vi "Generate waveform.vi"(8 "error in (no error)":errorcluster, 11 "Galvo in":refnum<class "InVivo_ImagingModeSPIM.lvclass">) -> (0 "error out":errorcluster, 2 "Array":variant[](array[variant]), 3 "Galvo out":refnum<class "InVivo_ImagingModeSPIM.lvclass">)   [LabVIEW 2012, in "InVivo_ImagingModeSPIM.lvclass"]
uses:
  InVivo_ImagingModeSPIM.lvclass
  InVivo_ImagingModeSPIM.lvclass/InVivo_ImagingModeSPIM.ctl
  <vilib>/measure/NI_MABase.lvlib
panel:
  out "Waveformvalues":variant
  out "Mixed Signal Graph 2":waveform(dbl)(graph)
  out "Mixed Signal Graph":waveform(dbl)[](graph)
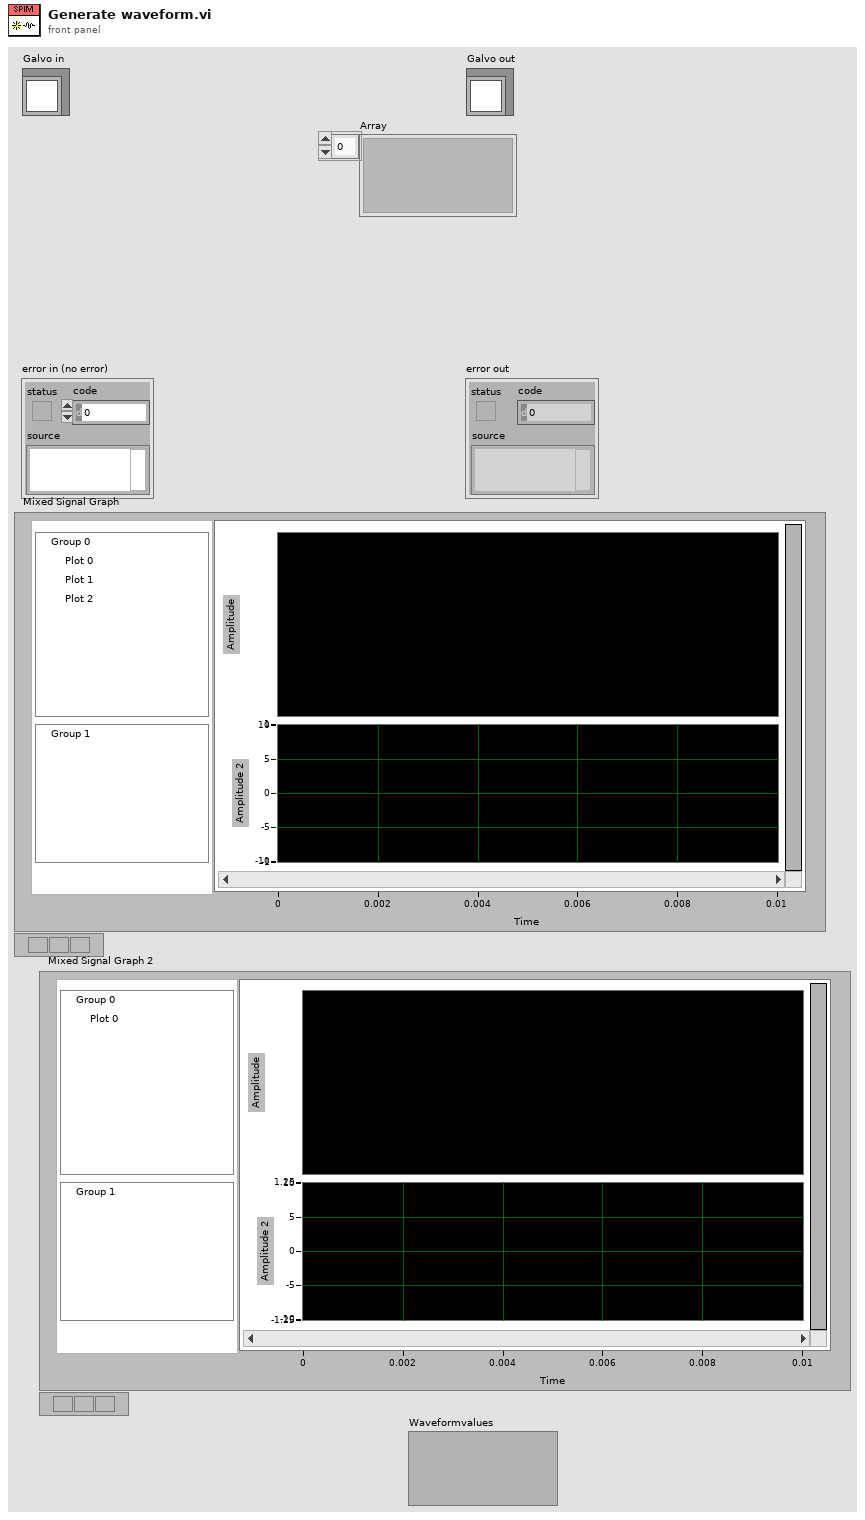
[diagram p1: front panel]
types:
  T1 = typedef "InVivo_ImagingModeSPIM.lvclass/waveform_enum.ctl" = enum16{"triangular", "sawtooth", "sinusodial"}
  T2 = typedef "InVivo_ImagingModeSPIM.lvclass/Control 4.ctl" = enum16{"Triangular", "Sawtooth", "Sinusoidal"}
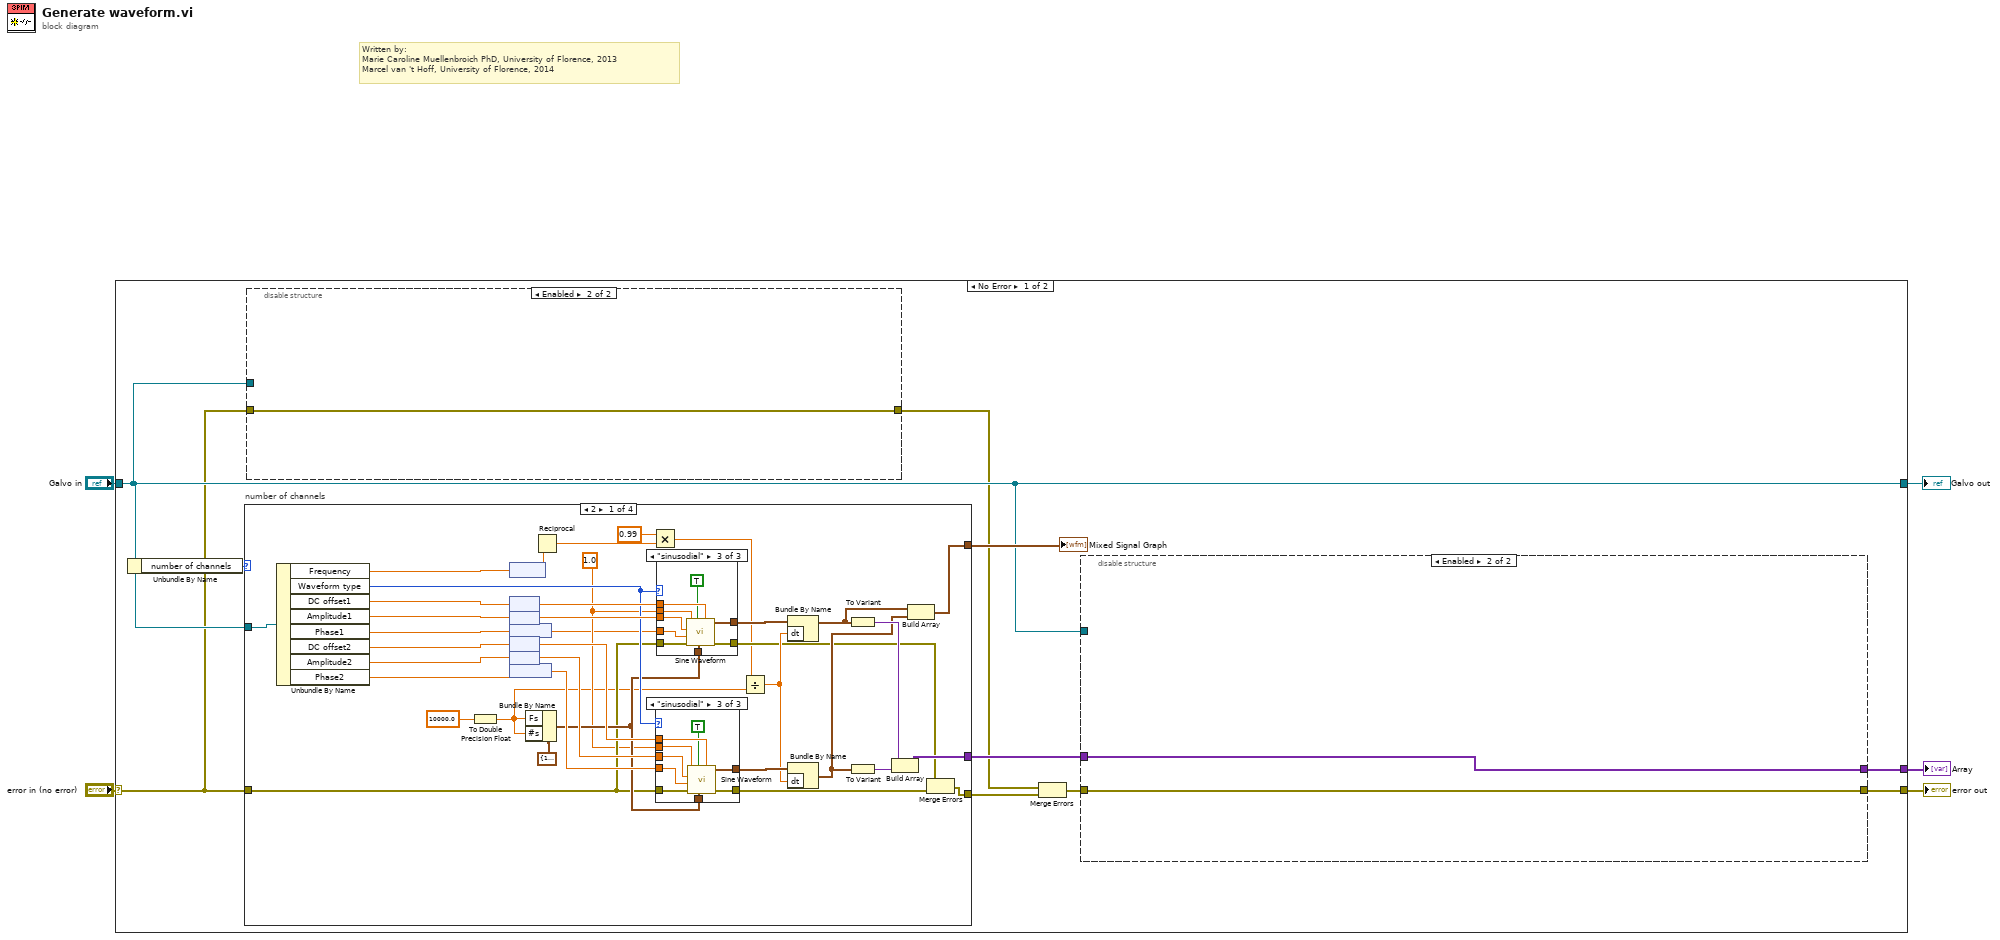
[diagram p0: block diagram]
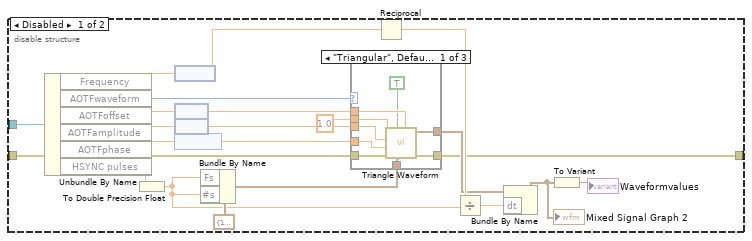
[diagram p2: hidden frame]
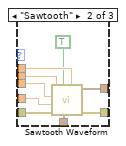
[diagram p3: hidden frame]
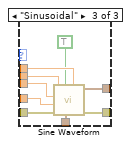
[diagram p4: hidden frame]
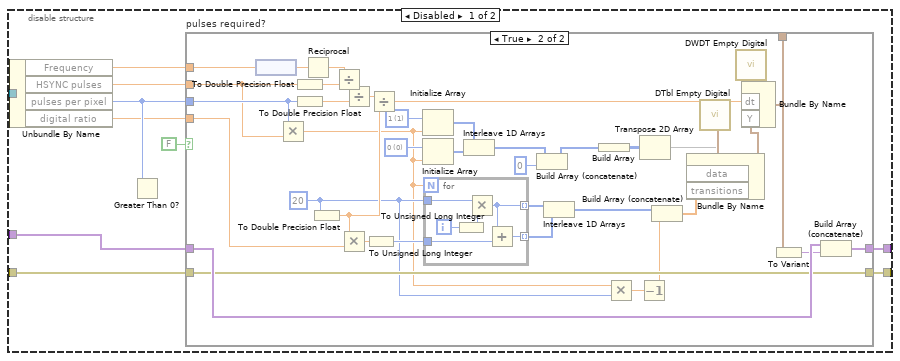
[diagram p5: hidden frame]
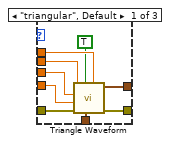
[diagram p7: hidden frame]
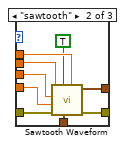
[diagram p8: hidden frame]
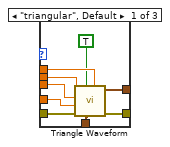
[diagram p9: hidden frame]
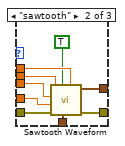
[diagram p10: hidden frame]
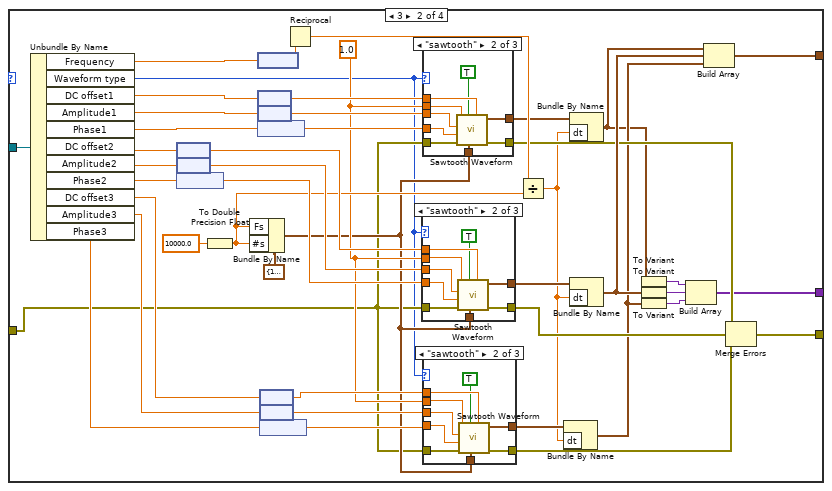
[diagram p11: hidden frame]
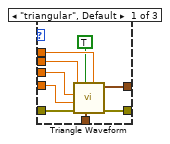
[diagram p12: hidden frame]
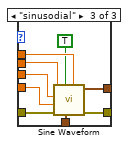
[diagram p13: hidden frame]
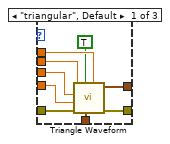
[diagram p14: hidden frame]
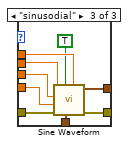
[diagram p15: hidden frame]
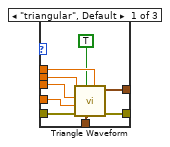
[diagram p16: hidden frame]
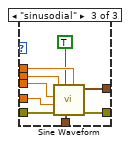
[diagram p17: hidden frame]
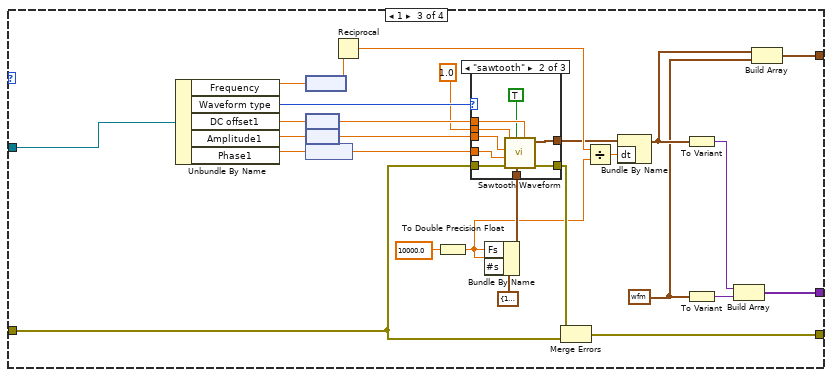
[diagram p18: hidden frame]
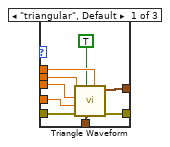
[diagram p19: hidden frame]
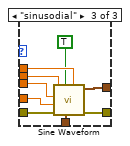
[diagram p20: hidden frame]
diagram:
  # "Written by:\nMarie Caroline Muellenbroich PhD, University of Florence, 2013 \nMarcel van 't Hoff, University of Florence, 2014"
  n1 = case shown="No Error" "error in (no error)" {
    selector: "error in (no error)" -> [w9 w398]
    tunnel: [w13 w398] -> w5
    tunnel: [w10 w397] -> w4
    tunnel: "Galvo in" -> [w10 w397]
    tunnel: [w15 _] -> w3
    frame No Error {
      n2 = Unbundle By Name(w10) -> ("number of channels"=w12:u8)
      n3 = case "number of channels" shown="2" w12 {
        tunnel: [w146 w223 w360 w396] -> w8
        tunnel: w9 -> [w147 w219 w346 w396]
        tunnel: [w145 w221 w359 _] -> w14
        tunnel: [w132 w222 w349 _] -> w11
        tunnel: w10 -> [w129 w220 w344 _]
        frame 2 {
          w141 = 1.0
          n4 = Unbundle By Name(w129) -> ("Frequency"=w138:dbl[unit], "Waveform type"=w155:T1, "DC offset1"=w156:dbl[unit], "Amplitude1"=w157:dbl[unit], "Phase1"=w158:dbl[unit], "DC offset2"=w153:dbl[unit], "Amplitude2"=w152:dbl[unit], "Phase2"=w151:dbl[unit])
          n5 = To Double Precision Float(number=10000.0) -> (double precision float=w136:dbl)
          n6 = node(w138) -> (w140:dbl)
          n7 = node(w156) -> (w160:dbl)
          n8 = node(w157) -> (w161:dbl)
          n9 = node(w158) -> (w137:dbl)
          n10 = node(w153) -> (w154:dbl)
          n11 = node(w152) -> (w149:dbl)
          n12 = node(w151) -> (w150:dbl)
          n13 = Bundle By Name(cluster=cluster{"Fs":dbl, "#s":dbl} {"Fs"=1000.0, "#s"=1000.0} ("sampling info"), "Fs"=w136, "#s"=w136) -> (w148:cluster{"Fs":dbl, "#s":dbl})
          n14 = Reciprocal(x=w140) -> (1/x=w127:dbl)
          n15 = Multiply(x=0.99, y=w127) -> (x*y=w126:dbl)
          n16 = case shown="\"sinusodial\"" w155 {
            tunnel: w154 -> [w168 w179 w188]
            tunnel: w141 -> [w167 w178 w187]
            tunnel: w148 -> [w169 w177 w186]
            tunnel: [w166 w176 w185] -> w139
            tunnel: [w170 w171 w180] -> w142
            tunnel: w149 -> [w163 w174 w183]
            tunnel: w150 -> [w164 w173 w182]
            tunnel: w147 -> [w162 w172 w181]
            frame "triangular", Default {
              n17 = call <vilib>:"Triangle Waveform.vi"("offset"=w168, "sampling info"=w169, "reset signal"=TRUE, "error in (no error)"=w162, "phase"=w164, "amplitude"=w163, "frequency"=w167) -> ("error out"=w170:errorcluster, "signal out"=w166:waveform(dbl))  [unwired: 3 in]
            }
            frame "sawtooth" {
              n18 = call <vilib>:"Sawtooth Waveform.vi"("offset"=w179, "sampling info"=w177, "reset signal"=TRUE, "error in (no error)"=w172, "phase"=w173, "amplitude"=w174, "frequency"=w178) -> ("error out"=w171:errorcluster, "signal out"=w176:waveform(dbl))  [unwired: 3 in]
            }
            frame "sinusodial" {
              n19 = call <vilib>:"Sine Waveform.vi"("offset"=w188, "sampling info"=w186, "reset signal"=TRUE, "error in (no error)"=w181, "phase"=w182, "amplitude"=w183, "frequency"=w187) -> ("error out"=w180:errorcluster, "signal out"=w185:waveform(dbl))  [unwired: 3 in]
            }
          }
          n20 = case shown="\"sinusodial\"" w155 {
            tunnel: w160 -> [w195 w206 w215]
            tunnel: w141 -> [w194 w205 w214]
            tunnel: w161 -> [w193 w204 w213]
            tunnel: w137 -> [w192 w203 w212]
            tunnel: w148 -> [w196 w202 w211]
            tunnel: [w191 w201 w210] -> w133
            tunnel: [w197 w200 w209] -> w130
            tunnel: w147 -> [w189 w198 w207]
            frame "triangular", Default {
              n21 = call <vilib>:"Triangle Waveform.vi"("offset"=w195, "sampling info"=w196, "reset signal"=TRUE, "error in (no error)"=w189, "phase"=w192, "amplitude"=w193, "frequency"=w194) -> ("error out"=w197:errorcluster, "signal out"=w191:waveform(dbl))  [unwired: 3 in]
            }
            frame "sawtooth" {
              n22 = call <vilib>:"Sawtooth Waveform.vi"("offset"=w206, "sampling info"=w202, "reset signal"=TRUE, "error in (no error)"=w198, "phase"=w203, "amplitude"=w204, "frequency"=w205) -> ("error out"=w200:errorcluster, "signal out"=w201:waveform(dbl))  [unwired: 3 in]
            }
            frame "sinusodial" {
              n23 = call <vilib>:"Sine Waveform.vi"("offset"=w215, "sampling info"=w211, "reset signal"=TRUE, "error in (no error)"=w207, "phase"=w212, "amplitude"=w213, "frequency"=w214) -> ("error out"=w209:errorcluster, "signal out"=w210:waveform(dbl))  [unwired: 3 in]
            }
          }
          n24 = Divide(x=w126, y=w136) -> (x/y=w135:dbl)
          n25 = Bundle By Name(cluster=w133, "dt"=w135) -> (w131:waveform(dbl))
          n26 = Bundle By Name(cluster=w139, "dt"=w135) -> (w134:waveform(dbl))
          n27 = To Variant(anything=w131) -> (Variant=w143:variant)
          n28 = To Variant(anything=w134) -> (Variant=w144:variant)
          n29 = Build Array(w143, w144) -> (w145:variant[])
          n30 = Build Array(w131, w134) -> (w132:waveform(dbl)[])
          n31 = Merge Errors(w130, w142) -> (w146:errorcluster)
        }
        frame 3 {
          w230 = 1.0
          n32 = Unbundle By Name(w220) -> ("Frequency"=w243:dbl[unit], "Waveform type"=w218:T1, "DC offset1"=w255:dbl[unit], "Amplitude1"=w256:dbl[unit], "Phase1"=w257:dbl[unit], "DC offset2"=w253:dbl[unit], "Amplitude2"=w252:dbl[unit], "Phase2"=w251:dbl[unit], "DC offset3"=w236:dbl[unit], "Amplitude3"=w235:dbl[unit], "Phase3"=w234:dbl[unit])
          n33 = node(w253) -> (w254:dbl)
          n34 = node(w252) -> (w249:dbl)
          n35 = node(w251) -> (w250:dbl)
          n36 = To Double Precision Float(number=10000.0) -> (double precision float=w241:dbl)
          n37 = Bundle By Name(cluster=cluster{"Fs":dbl, "#s":dbl} {"Fs"=1000.0, "#s"=1000.0} ("sampling info"), "Fs"=w241, "#s"=w241) -> (w229:cluster{"Fs":dbl, "#s":dbl})
          n38 = node(w243) -> (w245:dbl)
          n39 = node(w255) -> (w259:dbl)
          n40 = node(w256) -> (w260:dbl)
          n41 = node(w257) -> (w242:dbl)
          n42 = node(w236) -> (w233:dbl)
          n43 = node(w235) -> (w232:dbl)
          n44 = node(w234) -> (w231:dbl)
          n45 = Reciprocal(x=w245) -> (1/x=w240:dbl)
          n46 = case shown="\"sawtooth\"" w218 {
            tunnel: w254 -> [w294 w305 w314]
            tunnel: w230 -> [w293 w304 w313]
            tunnel: w229 -> [w295 w303 w312]
            tunnel: [w292 w302 w311] -> w244
            tunnel: [w296 w297 w306] -> w246
            tunnel: w249 -> [w289 w300 w309]
            tunnel: w250 -> [w290 w299 w308]
            tunnel: w219 -> [w288 w298 w307]
            frame "triangular", Default {
              n47 = call <vilib>:"Triangle Waveform.vi"("offset"=w294, "sampling info"=w295, "reset signal"=TRUE, "error in (no error)"=w288, "phase"=w290, "amplitude"=w289, "frequency"=w293) -> ("error out"=w296:errorcluster, "signal out"=w292:waveform(dbl))  [unwired: 3 in]
            }
            frame "sawtooth" {
              n48 = call <vilib>:"Sawtooth Waveform.vi"("offset"=w305, "sampling info"=w303, "reset signal"=TRUE, "error in (no error)"=w298, "phase"=w299, "amplitude"=w300, "frequency"=w304) -> ("error out"=w297:errorcluster, "signal out"=w302:waveform(dbl))  [unwired: 3 in]
            }
            frame "sinusodial" {
              n49 = call <vilib>:"Sine Waveform.vi"("offset"=w314, "sampling info"=w312, "reset signal"=TRUE, "error in (no error)"=w307, "phase"=w308, "amplitude"=w309, "frequency"=w313) -> ("error out"=w306:errorcluster, "signal out"=w311:waveform(dbl))  [unwired: 3 in]
            }
          }
          n50 = case shown="\"sawtooth\"" w218 {
            tunnel: w259 -> [w321 w332 w341]
            tunnel: w230 -> [w320 w331 w340]
            tunnel: w260 -> [w319 w330 w339]
            tunnel: w242 -> [w318 w329 w338]
            tunnel: w229 -> [w322 w328 w337]
            tunnel: [w317 w327 w336] -> w238
            tunnel: [w323 w326 w335] -> w237
            tunnel: w219 -> [w315 w324 w333]
            frame "triangular", Default {
              n51 = call <vilib>:"Triangle Waveform.vi"("offset"=w321, "sampling info"=w322, "reset signal"=TRUE, "error in (no error)"=w315, "phase"=w318, "amplitude"=w319, "frequency"=w320) -> ("error out"=w323:errorcluster, "signal out"=w317:waveform(dbl))  [unwired: 3 in]
            }
            frame "sawtooth" {
              n52 = call <vilib>:"Sawtooth Waveform.vi"("offset"=w332, "sampling info"=w328, "reset signal"=TRUE, "error in (no error)"=w324, "phase"=w329, "amplitude"=w330, "frequency"=w331) -> ("error out"=w326:errorcluster, "signal out"=w327:waveform(dbl))  [unwired: 3 in]
            }
            frame "sinusodial" {
              n53 = call <vilib>:"Sine Waveform.vi"("offset"=w341, "sampling info"=w337, "reset signal"=TRUE, "error in (no error)"=w333, "phase"=w338, "amplitude"=w339, "frequency"=w340) -> ("error out"=w335:errorcluster, "signal out"=w336:waveform(dbl))  [unwired: 3 in]
            }
          }
          n54 = case shown="\"sawtooth\"" w218 {
            tunnel: w233 -> [w267 w278 w287]
            tunnel: w230 -> [w266 w277 w286]
            tunnel: w229 -> [w268 w276 w285]
            tunnel: [w265 w275 w284] -> w228
            tunnel: [w269 w270 w279] -> w227
            tunnel: w232 -> [w262 w273 w282]
            tunnel: w231 -> [w263 w272 w281]
            tunnel: w219 -> [w261 w271 w280]
            frame "triangular", Default {
              n55 = call <vilib>:"Triangle Waveform.vi"("offset"=w267, "sampling info"=w268, "reset signal"=TRUE, "error in (no error)"=w261, "phase"=w263, "amplitude"=w262, "frequency"=w266) -> ("error out"=w269:errorcluster, "signal out"=w265:waveform(dbl))  [unwired: 3 in]
            }
            frame "sawtooth" {
              n56 = call <vilib>:"Sawtooth Waveform.vi"("offset"=w278, "sampling info"=w276, "reset signal"=TRUE, "error in (no error)"=w271, "phase"=w272, "amplitude"=w273, "frequency"=w277) -> ("error out"=w270:errorcluster, "signal out"=w275:waveform(dbl))  [unwired: 3 in]
            }
            frame "sinusodial" {
              n57 = call <vilib>:"Sine Waveform.vi"("offset"=w287, "sampling info"=w285, "reset signal"=TRUE, "error in (no error)"=w280, "phase"=w281, "amplitude"=w282, "frequency"=w286) -> ("error out"=w279:errorcluster, "signal out"=w284:waveform(dbl))  [unwired: 3 in]
            }
          }
          n58 = Divide(x=w240, y=w241) -> (x/y=w226:dbl)
          n59 = Bundle By Name(cluster=w228, "dt"=w226) -> (w224:waveform(dbl))
          n60 = Bundle By Name(cluster=w238, "dt"=w226) -> (w216:waveform(dbl))
          n61 = Bundle By Name(cluster=w244, "dt"=w226) -> (w239:waveform(dbl))
          n62 = To Variant(anything=w216) -> (Variant=w247:variant)
          n63 = To Variant(anything=w239) -> (Variant=w248:variant)
          n64 = To Variant(anything=w224) -> (Variant=w225:variant)
          n65 = Build Array(w247, w248, w225) -> (w221:variant[])
          n66 = Build Array(w216, w239, w224) -> (w222:waveform(dbl)[])
          n67 = Merge Errors(w237, w246, w227) -> (w223:errorcluster)
        }
        frame 1 {
          w345 = waveform(dbl) {"t0"=timestamp(0 s since 1904-01-01), "dt"=1.0, "Y"=[]} ("signal out")
          n68 = Unbundle By Name(w344) -> ("Frequency"=w354:dbl[unit], "Waveform type"=w362:T1, "DC offset1"=w363:dbl[unit], "Amplitude1"=w364:dbl[unit], "Phase1"=w365:dbl[unit])
          n69 = node(w354) -> (w355:dbl)
          n70 = node(w363) -> (w367:dbl)
          n71 = node(w364) -> (w368:dbl)
          n72 = node(w365) -> (w353:dbl)
          n73 = Reciprocal(x=w355) -> (1/x=w352:dbl)
          n74 = To Double Precision Float(number=10000.0) -> (double precision float=w342:dbl)
          n75 = Bundle By Name(cluster=cluster{"Fs":dbl, "#s":dbl} {"Fs"=10000.0, "#s"=10000.0} ("sampling info"), "Fs"=w342, "#s"=w342) -> (w361:cluster{"Fs":dbl, "#s":dbl})
          n76 = case shown="\"sawtooth\"" w362 {
            tunnel: w367 -> [w375 w386 w395]
            tunnel: 1.0 -> [w374 w385 w394]
            tunnel: w368 -> [w373 w384 w393]
            tunnel: w353 -> [w372 w383 w392]
            tunnel: w361 -> [w376 w382 w391]
            tunnel: [w371 w381 w390] -> w350
            tunnel: [w377 w380 w389] -> w347
            tunnel: w346 -> [w369 w378 w387]
            frame "triangular", Default {
              n77 = call <vilib>:"Triangle Waveform.vi"("offset"=w375, "sampling info"=w376, "reset signal"=TRUE, "error in (no error)"=w369, "phase"=w372, "amplitude"=w373, "frequency"=w374) -> ("error out"=w377:errorcluster, "signal out"=w371:waveform(dbl))  [unwired: 3 in]
            }
            frame "sawtooth" {
              n78 = call <vilib>:"Sawtooth Waveform.vi"("offset"=w386, "sampling info"=w382, "reset signal"=TRUE, "error in (no error)"=w378, "phase"=w383, "amplitude"=w384, "frequency"=w385) -> ("error out"=w380:errorcluster, "signal out"=w381:waveform(dbl))  [unwired: 3 in]
            }
            frame "sinusodial" {
              n79 = call <vilib>:"Sine Waveform.vi"("offset"=w395, "sampling info"=w391, "reset signal"=TRUE, "error in (no error)"=w387, "phase"=w392, "amplitude"=w393, "frequency"=w394) -> ("error out"=w389:errorcluster, "signal out"=w390:waveform(dbl))  [unwired: 3 in]
            }
          }
          n80 = Merge Errors(w347, w346) -> (w360:errorcluster)
          n81 = Divide(x=w352, y=w342) -> (x/y=w351:dbl)
          n82 = Bundle By Name(cluster=w350, "dt"=w351) -> (w348:waveform(dbl))
          n83 = To Variant(anything=w348) -> (Variant=w357:variant)
          n84 = To Variant(anything=w345) -> (Variant=w358:variant)
          n85 = Build Array(w357, w358) -> (w359:variant[])
          n86 = Build Array(w348, w345) -> (w349:waveform(dbl)[])
        }
        frame Default {
        }
      }
      "Mixed Signal Graph" <- w11
      n87 = disable-structure shown="Enabled" {
        disable-tunnel: w10 -> [w37 _]
        disable-tunnel: w9 -> [w36 w65]
        disable-tunnel: [w17 w65] -> w6
        frame Disabled {
          n88 = Unbundle By Name(w37) -> ("Frequency"=w23:dbl[unit], "AOTFwaveform"=w28:T2, "AOTFoffset"=w29:dbl[unit], "AOTFamplitude"=w30:dbl[unit], "AOTFphase"=w31:dbl[unit], "HSYNC pulses"=w27:dbl)
          n89 = To Double Precision Float(number=w27) -> (double precision float=w21:dbl)
          n90 = node(w23) -> (w24:dbl)
          n91 = node(w29) -> (w33:dbl)
          n92 = node(w30) -> (w34:dbl)
          n93 = node(w31) -> (w22:dbl)
          n94 = Bundle By Name(cluster=cluster{"Fs":dbl, "#s":dbl} {"Fs"=1000.0, "#s"=1000.0} ("sampling info"), "Fs"=w21, "#s"=w21) -> (w26:cluster{"Fs":dbl, "#s":dbl})
          n95 = case shown="\"Triangular\", Default" w28 {
            tunnel: w33 -> [w44 w55 w64]
            tunnel: 1.0 -> [w43 w54 w63]
            tunnel: w34 -> [w42 w53 w62]
            tunnel: w22 -> [w41 w52 w61]
            tunnel: w26 -> [w45 w51 w60]
            tunnel: [w40 w50 w59] -> w18
            tunnel: [w46 w49 w58] -> w17
            tunnel: w36 -> [w38 w47 w56]
            frame "Triangular", Default {
              n96 = call <vilib>:"Triangle Waveform.vi"("offset"=w44, "sampling info"=w45, "reset signal"=TRUE, "error in (no error)"=w38, "phase"=w41, "amplitude"=w42, "frequency"=w43) -> ("error out"=w46:errorcluster, "signal out"=w40:waveform(dbl))  [unwired: 3 in]
            }
            frame "Sawtooth" {
              n97 = call <vilib>:"Sawtooth Waveform.vi"("offset"=w55, "sampling info"=w51, "reset signal"=TRUE, "error in (no error)"=w47, "phase"=w52, "amplitude"=w53, "frequency"=w54) -> ("error out"=w49:errorcluster, "signal out"=w50:waveform(dbl))  [unwired: 3 in]
            }
            frame "Sinusoidal" {
              n98 = call <vilib>:"Sine Waveform.vi"("offset"=w64, "sampling info"=w60, "reset signal"=TRUE, "error in (no error)"=w56, "phase"=w61, "amplitude"=w62, "frequency"=w63) -> ("error out"=w58:errorcluster, "signal out"=w59:waveform(dbl))  [unwired: 3 in]
            }
          }
          n99 = Reciprocal(x=w24) -> (1/x=w20:dbl)
          n100 = Divide(x=w20, y=w21) -> (x/y=w19:dbl)
          n101 = Bundle By Name(cluster=w18, "dt"=w19) -> (w16:waveform(dbl))
          "Mixed Signal Graph 2" <- w16
          n102 = To Variant(anything=w16) -> (Variant=→"Waveformvalues":variant)
        }
        frame Enabled {
        }
      }
      n103 = Merge Errors(w6, w8) -> (w7:errorcluster)
      n104 = disable-structure shown="Enabled" {
        disable-tunnel: [w75 w123] -> w15
        disable-tunnel: w14 -> [w74 w123]
        disable-tunnel: [w70 w124] -> w13
        disable-tunnel: w10 -> [w67 _]
        disable-tunnel: w7 -> [w66 w124]
        frame Disabled {
          n105 = Unbundle By Name(w67) -> ("Frequency"=w73:dbl[unit], "HSYNC pulses"=w72:dbl, "pulses per pixel"=w71:i32, "digital ratio"=w69:dbl)
          n106 = Greater Than 0?(x=w71) -> ()  [unwired: 1 out]
          n107 = case "pulses required?" shown="True" FALSE {
            tunnel: w71 -> [_ w81]
            tunnel: [w77 w98] -> w70
            tunnel: w66 -> [w77 w98]
            tunnel: [w76 w111] -> w75
            tunnel: w74 -> [w76 w112]
            tunnel: w73 -> [_ w116]
            tunnel: w72 -> [_ w78]
            tunnel: [_ w108] -> _
            tunnel: w69 -> [_ w94]
            frame False {
            }
            frame True {
              w82 = u32 20 ("ratio step size")
              w100 = u8 0 items=["0", "1", "Z", "L", "H", "X", "T", "V"] ("value 2")
              w99 = u8 1 items=["0", "1", "Z", "L", "H", "X", "T", "V"] ("value 2")
              n108 = node(w116) -> (w115:dbl)
              n109 = Multiply(x=w81, y=w78) -> (x*y=w79:dbl)
              n110 = To Double Precision Float(number=w78) -> (double precision float=w113:dbl)
              n111 = To Double Precision Float(number=w81) -> (double precision float=w109:dbl)
              n112 = Reciprocal(x=w115) -> (1/x=w114:dbl)
              n113 = To Double Precision Float(number=w82) -> (double precision float=w93:dbl)
              n114 = Divide(x=w114, y=w113) -> (x/y=w110:dbl)
              n115 = Multiply(x=w93, y=w94) -> (x*y=w104:dbl)
              n116 = Divide(x=w110, y=w109) -> (x/y=w92:dbl)
              n117 = To Unsigned Long Integer(number=w104) -> (unsigned 32bit integer=w107:u32)
              n118 = Divide(x=w92, y=w93) -> (x/y=w91:dbl)
              n119 = Initialize Array(w99, w79) -> (w102:u8[])
              n120 = Initialize Array(w100, w79) -> (w103:u8[])
              n121 = for {
                N: w79 -> [_]
                tunnel: w107 -> [w120]
                tunnel: w82 -> [w122]
                tunnel: [w119] -> w105 mode=indexing
                tunnel: [w118] -> w106 mode=indexing
                i -> [w121]
                n122 = To Unsigned Long Integer(number=w121) -> (unsigned 32bit integer=w117:u32)
                n123 = Multiply(x=w122, y=w117) -> (x*y=w119:u32)
                n124 = Add(x=w119, y=w120) -> (x+y=w118:u32)
              }
              n125 = Interleave 1D Arrays(w102, w103) -> (w87:u8[])
              n126 = Build Array (concatenate)(w87, u8 0 ("value 2")) -> (w86:u8[])
              n127 = Interleave 1D Arrays(w105, w106) -> (w85:u32[])
              n128 = Build Array(w86) -> (w101:u8[][])
              n129 = Multiply(x=w79, y=w82) -> (x*y=w83:dbl)
              n130 = Decrement(x=w83) -> (x-1=w80:dbl)
              n131 = Transpose 2D Array(2D array=w101) -> (transposed array=w89:u8[][])
              n132 = Build Array (concatenate)(w85, w80) -> (w84:dbl[])
              n133 = call <vilib>:"DTbl Empty Digital.vi"() -> ("digital data"=w97:digitaldata)  [unwired: 5 in]
              n134 = Bundle By Name(cluster=w97, "data"=w89, "transitions"=w84) -> (w95:digitaldata)
              n135 = call <vilib>:"DWDT Empty Digital.vi"() -> ("digital waveform out"=w96:digitalwaveform)  [unwired: 5 in]
              n136 = Bundle By Name(cluster=w96, "dt"=w91, "Y"=w95) -> (w108:digitalwaveform)
              n137 = To Variant(anything=w108) -> (Variant=w90:variant)
              n138 = Build Array (concatenate)(w112, w90) -> (w111:variant[])
            }
          }
        }
        frame Enabled {
        }
      }
    }
    frame Error {
    }
  }
  "error out" <- w5
  "Galvo out" <- w4
  "Array" <- w3
